vi "CLC_Power_InPhase_Cal_Channel.vi"(8 "error in":errorcluster, 11 "Channel IN":i32=16) -> (0 "error out":errorcluster, 1 "Channel":i32, 3 "Ref_Channel":i32)   [LabVIEW 2023]
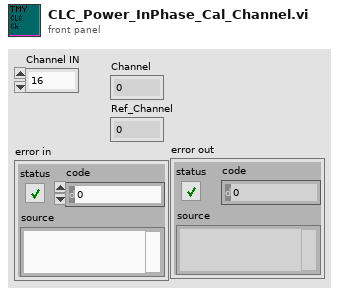
[diagram p1: front panel]
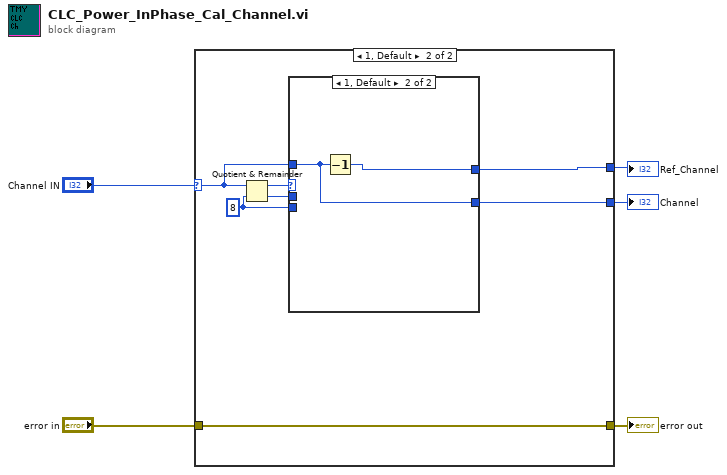
[diagram p0: block diagram]
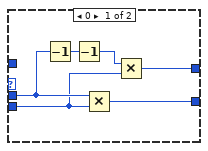
[diagram p3: hidden frame]
diagram:
  n1 = case shown="1, Default" "Channel IN" {
    selector: "Channel IN" -> [w6 w10]
    tunnel: [w6 w11] -> w4
    tunnel: [w6 w8] -> w5
    tunnel: "error in" -> [w7 w9]
    tunnel: [w7 w9] -> w1
    frame 0 {
    }
    frame 1, Default {
      w12 = 8 ("y")
      n2 = Quotient & Remainder(x=w10, y=w12) -> (x-y*floor(x/y)=w14:i32, floor(x/y)=w13:i32)
      n3 = case shown="1, Default" w14 {
        tunnel: w13 -> [w17 _]
        tunnel: w12 -> [w16 _]
        tunnel: [w20 w22] -> w11
        tunnel: [w18 w21] -> w8
        tunnel: w10 -> [_ w22]
        frame 0 {
          n4 = Decrement(x=w17) -> (x-1=w15:i32)
          n5 = Decrement(x=w15) -> (x-1=w19:i32)
          n6 = Multiply(x=w17, y=w16) -> (x*y=w20:i32)
          n7 = Multiply(x=w19, y=w16) -> (x*y=w18:i32)
        }
        frame 1, Default {
          n8 = Decrement(x=w22) -> (x-1=w21:i32)
        }
      }
    }
  }
  "Channel" <- w4
  "Ref_Channel" <- w5
  "error out" <- w1
